vi "Read_Preproc_File_Path.vi"(8 "error in (no error)":errorcluster, 11 "Python in":refnum<class "Python.lvclass">) -> (0 "error out":errorcluster, 2 "File_Path":path, 3 "Python out":refnum<class "Python.lvclass">)   [LabVIEW 2020, in "Python.lvclass"]
uses:
  Python.lvclass
  Python.lvclass/Python.ctl
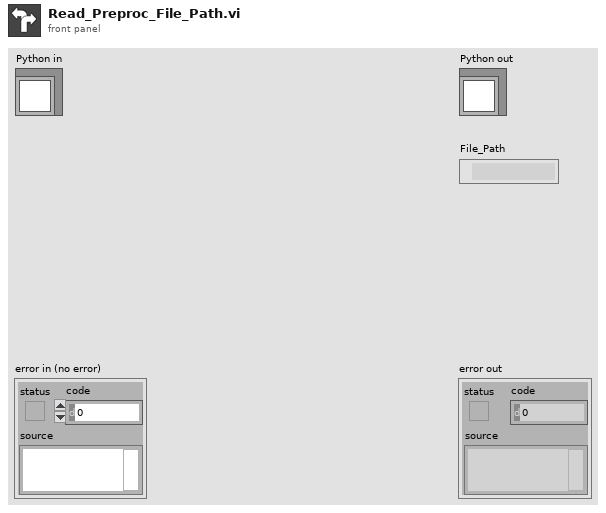
[diagram p1: front panel]
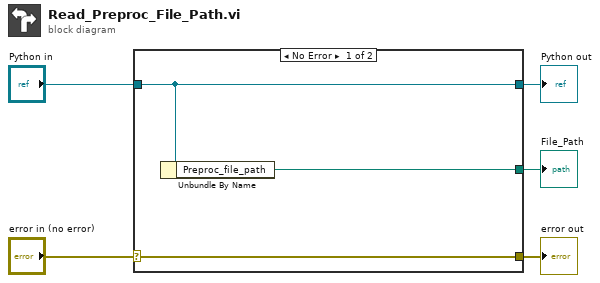
[diagram p0: block diagram]
diagram:
  n1 = case shown="No Error" "error in (no error)" {
    selector: "error in (no error)" -> [w8 w9]
    tunnel: [w8 w9] -> w4
    tunnel: [w7 w10] -> w2
    tunnel: "Python in" -> [w7 w10]
    tunnel: [w6 _] -> w1
    frame No Error {
      n2 = Unbundle By Name(w7) -> ("Preproc_file_path"=w6:path)
    }
    frame Error {
    }
  }
  "error out" <- w4
  "Python out" <- w2
  "File_Path" <- w1
